vi "Polynomial Error code global.vi"() -> ()   [LabVIEW 2018, in "NI_AALPro.lvlib"]
uses:
  NI_AALPro.lvlib
panel:
  in  "MatrixInfNanErr":i32=-20068
  in  "DimensionErr":i32=-20058
  in  "start>end":i32=-20104
  in  "end is root":i32=-20103
  in  "start is root":i32=-20102
  in  "coef. of poly are all zero":i32=-20101
  in  "minus order":i32=-20021
  in  "not a square matrix":i32=-20040
  in  "divide by zero":i32=-20060
  in  "empty array":i32=20003
  # "for Create Orthogonal Poly"
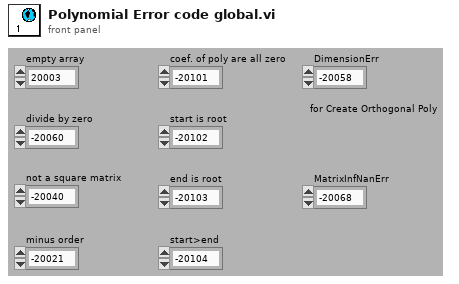
[diagram p1: front panel]
diagram:
